vi "add_SetSonarLights.vi"(4 "Lights":T1, 5 "msg in":string) -> (2 "msg out":string)   [LabVIEW 2013]
uses:
  Primitives/subs/u16Scalar.vi
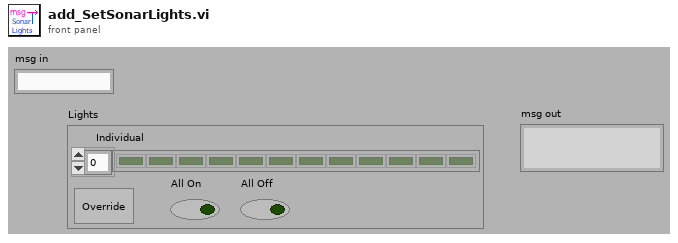
[diagram p1: front panel]
types:
  T1 = cluster{"Behavior":bool, "All On":bool, "All Off":bool, "Individual":bool[]}
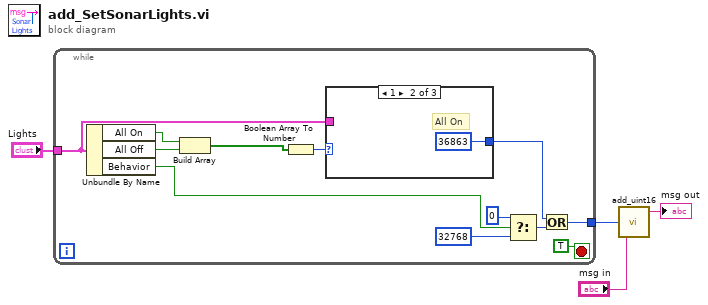
[diagram p0: block diagram]
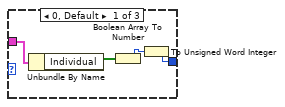
[diagram p2: hidden frame]
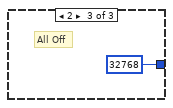
[diagram p3: hidden frame]
diagram:
  n1 = while {
    tunnel: "Lights" -> [w12]
    tunnel: [w6] -> w3
    stop <- TRUE stop-if-true
    n2 = Unbundle By Name(w12) -> ("All On"=w16:bool, "All Off"=w15:bool, "Behavior"=w11:bool)
    n3 = Build Array(w16, w15) -> (w5:bool[])
    n4 = Boolean Array To Number(Boolean array=w5) -> (number=w14:u32)
    n5 = case shown="1" w14 {
      tunnel: w12 -> [w20 _ _]
      tunnel: [w17 u16 36863 u16 32768 ("f")] -> w7
      frame 0, Default {
        n6 = Unbundle By Name(w20) -> ("Individual"=w19:bool[])
        n7 = Boolean Array To Number(Boolean array=w19) -> (number=w18:u32)
        n8 = To Unsigned Word Integer(number=w18) -> (unsigned 16bit integer=w17:u16)
      }
      frame 1 {
        # "All On"
      }
      frame 2 {
        # "All Off"
      }
    }
    n9 = Select(t=u16 0, s=w11, f=u16 32768) -> (s? t:f=w8:u16)
    n10 = Or(x=w7, y=w8) -> (x .or. y?=w6:u16)
  }
  n11 = call-poly "add_uint16.vi"("Numeric"=w3, "msg in"="msg in") -> ("msg out"=→"msg out":string)  [unwired: 3 in]
